vi "Execute.vi"(8 "error in (no error)":errorcluster, 10 "Abstract Producer in":refnum<class "Abstract Producer.lvclass">, 11 "Consumer Name Response Message in":refnum<class "Consumer Name Response Message.lvclass">) -> (0 "error out":errorcluster, 2 "Abstract Producer out":refnum<class "Abstract Producer.lvclass">, 3 "Consumer Name Response Message out":refnum<class "Consumer Name Response Message.lvclass">)   [LabVIEW 2017, in "Consumer Name Response Message.lvclass"]
uses:
  Consumer Name Response Message.lvclass
  Producer/Abstract Producer/Abstract Producer.lvclass
  Message List Action.ctl
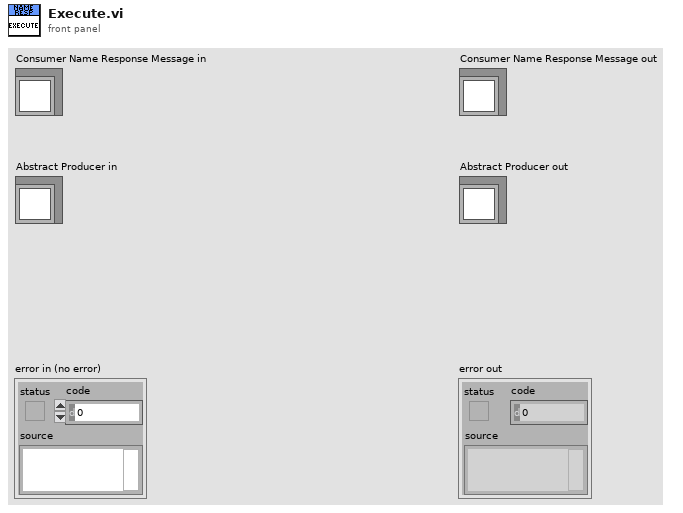
[diagram p1: front panel]
types:
  T1 = typedef "Message List Action.ctl" = enum16{"Get", "Add", "Reset"}
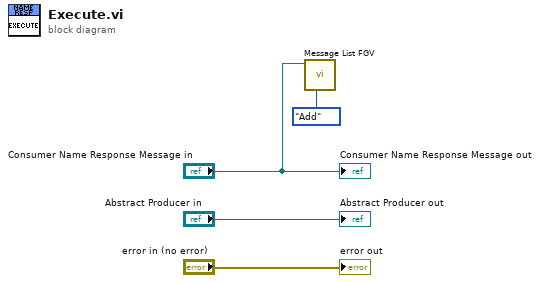
[diagram p0: block diagram]
diagram:
  n1 = call "Message List FGV.vi"("Action (Get)"=Message_List_Action."Add", "Message Object"="Consumer Name Response Message in") -> ()  [unwired: 8 in, 2 out]
  "error out" <- "error in (no error)"
  "Consumer Name Response Message out" <- "Consumer Name Response Message in"
  "Abstract Producer out" <- "Abstract Producer in"
